vi "pb_init.vi"(8 "error in (no error)":errorcluster, 11 "path in":path=path "C:/Program Files/SpinCore/SpinAPI/dll/spinapi.dll") -> (0 "error out":errorcluster, 3 "path out":path)   [LabVIEW 2018]
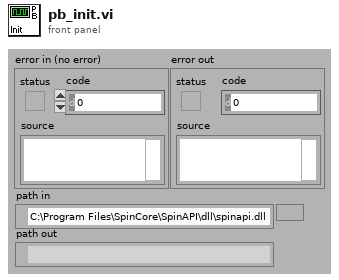
[diagram p1: front panel]
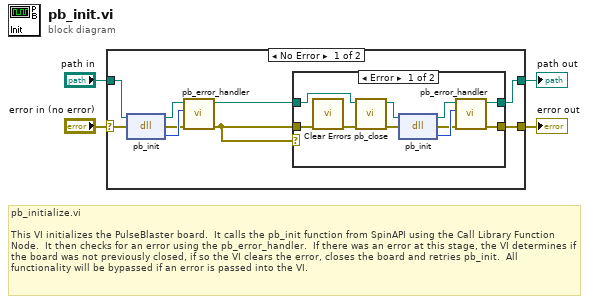
[diagram p0: block diagram]
diagram:
  # "pb_initialize.vi\n\nThis VI initializes the PulseBlaster board.  It calls the pb_init function from SpinAPI using the Call Library Function Node.  It then checks for an error using the pb_error_handler.  If there was an error at this stage, the VI determines if the board was not previously closed, if so the VI clears the error, closes the board and retries pb_init.  All functionality will be bypassed if an error is passed into the VI."
  n1 = case shown="No Error" "error in (no error)" {
    selector: "error in (no error)" -> [w12 w27]
    tunnel: [w8 w27] -> w4
    tunnel: [w7 w26] -> w2
    tunnel: "path in" -> [w6 w26]
    frame No Error {
      n2 = dll-call lib="C:/Program Files/SpinCore/SpinAPI/dll/spinapi.dll" fn="pb_init"(path in=w6, error in=w12) -> (path out=w11:path, error out=w10:errorcluster, "return type"=w13:i32)  [unwired: 1 in]
      n3 = call "pb_error_handler.vi"("error in (no error)"=w10, "return code"=w13, "path in"=w11) -> ("error out"=w5:errorcluster, "path out"=w9:path)  [unwired: 7 out]
      n4 = case shown="Error" w5 {
        tunnel: [w22 w24] -> w7
        tunnel: w5 -> [w21 w25]
        tunnel: w9 -> [w19 w24]
        tunnel: [w14 w25] -> w8
        frame Error {
          n5 = call <vilib>:"Clear Errors.vi"("error in (no error)"=w21) -> ("error out"=w20:errorcluster)  [unwired: 1 in, 5 out]
          n6 = call "pb_close.vi"("error in (no error)"=w20, "path in"=w19) -> ("error out"=w17:errorcluster, "path out"=w18:path)  [unwired: 8 out]
          n7 = dll-call lib="C:/Program Files/SpinCore/SpinAPI/dll/spinapi.dll" fn="pb_init"(path in=w18, error in=w17) -> (path out=w16:path, error out=w15:errorcluster, "return type"=w23:i32)  [unwired: 1 in]
          n8 = call "pb_error_handler.vi"("error in (no error)"=w15, "return code"=w23, "path in"=w16) -> ("error out"=w14:errorcluster, "path out"=w22:path)  [unwired: 7 out]
        }
        frame No Error {
        }
      }
    }
    frame Error {
    }
  }
  "error out" <- w4
  "path out" <- w2
